vi "挥发酚断电保存全局变量.vi"() -> ()   [LabVIEW 2022 SP3, in "挥发酚.lvlib"]
panel:
  in  "数据时间":T1
  in  "维护模式":bool
  in  "校准信息":T2
  in  "校准信息改变":bool
  in  "关键参数改变":bool
  in  "标样核查自动补测":bool caption="通讯连接"
  in  "跨度核查自动补测":bool caption="通讯连接"
  in  "零点核查自动补测":bool caption="通讯连接"
  out "校准条件":cluster{"线性相关系数":dbl}={"线性相关系数"=0.99}
  in  "CODMn关键参数":T3={"测量量程"=0.0, "测量检出限"=0.0, "测量精度"=0.0, "测量间隔"=0.0, "消解温度"=95.0, "消解时长"=25.0, "三项式系数"=0.0, "二次多项式系数"=0.0, "曲线斜率"=0.0, "曲线截距"=0.0, "线性相关系数"=0.0, "空白校准时间"=timestamp(0 s since 1904-01-01), "标样校准时间"=timestamp(0 s since 1904-01-01), "测量信号值"=0.0, "稀释倍数"=0.0, "量程系数"=0.0}
  in  "CODMn仪器参数":T4
  in  "阀口名称":T5={"V"="试剂1", "V 2"="试剂2", "V 3"="试剂3", "V 4"="试剂4", "V 5"="试剂5", "V 6"="试剂6", "V 7"="试剂7", "V 8"="试剂8", "V 9"="试剂9", "V 10"="试剂10", "V 11"="试剂11", "V 12"="试剂12", "V9-1"="试剂13", "V9-2"="试剂14"}
  out "阀配置":u8(ring) items=["三通阀", "排阀"]
  in  "远程标样校准":enum16{"标液1", "标液2", "标液3", "标液4"}(ring)
  in  "远程校准量程":enum16{"低量程1", "低量程2", "高量程1", "高量程2"}(ring)
  in  "站号":u16(ring)=1 items=["挥发酚"=1, "总氮"=2, "氨氮"=3]
  out "公式、校准输出":T6={"公式"={"X^2"=0.0, "X"=nan, "B"=nan}, "校准"={"校准？"=FALSE, "校准点1-5"=0, "校准浓度"=0.0}}
  in  "MB通信方式选择":enum16{"串口", "TCP"}(ring)
  in  "PORT":string="502"
  in  "IP":string="192.168.1.203"
  in  "VISA Resource":refnum<visa-resource-name>="COM4"
  in  "运行周期":T7={"运行模式"=enum."维护模式", "质控频次"=enum."关闭", "空白核查时间"=2, "跨度核查时间"=6, "测量间隔"=240} {"跨度核查时间" items=["00H", "01H", "02H", "03H", "04H", "05H", "06H", "07H", "08H", "09H", "10H", "11H", "12H", "13H", "14H", "15H", "16H", "17H", "18H", "19H", "20H", "21H", "22H", "23H", "关闭"]; "空白核查时间" items=["00H", "01H", "02H", "03H", "04H", "05H", "06H", "07H", "08H", "09H", "10H", "11H", "12H", "13H", "14H", "15H", "16H", "17H", "18H", "19H", "20H", "21H", "22H", "23H", "关闭"]}
  in  "流程路径":path=path "C:/Users/std/Documents/斯坦道流程文件/流程.xml"
  in  "质控参数设置":T8 {"标准液标准偏差" format="%#_g%"; "跨度标准液偏差" format="%#_g%"}
  # "运行模式："
  # "质控频次："
  # "零点核查时间："
  # "跨度核查时间："
  # "测量间隔："
  # "质控参数设置"
  # "监测参数"
  # "CODMn"
  # "跨度值"
  # "零点核查标准液浓度"
  # "跨度核查标准液浓度"
  # "标样核查标准液浓度"
  # "零点核查标准液偏差"
  # "跨度核查标准液偏差"
  # "标样核查标准液偏差"
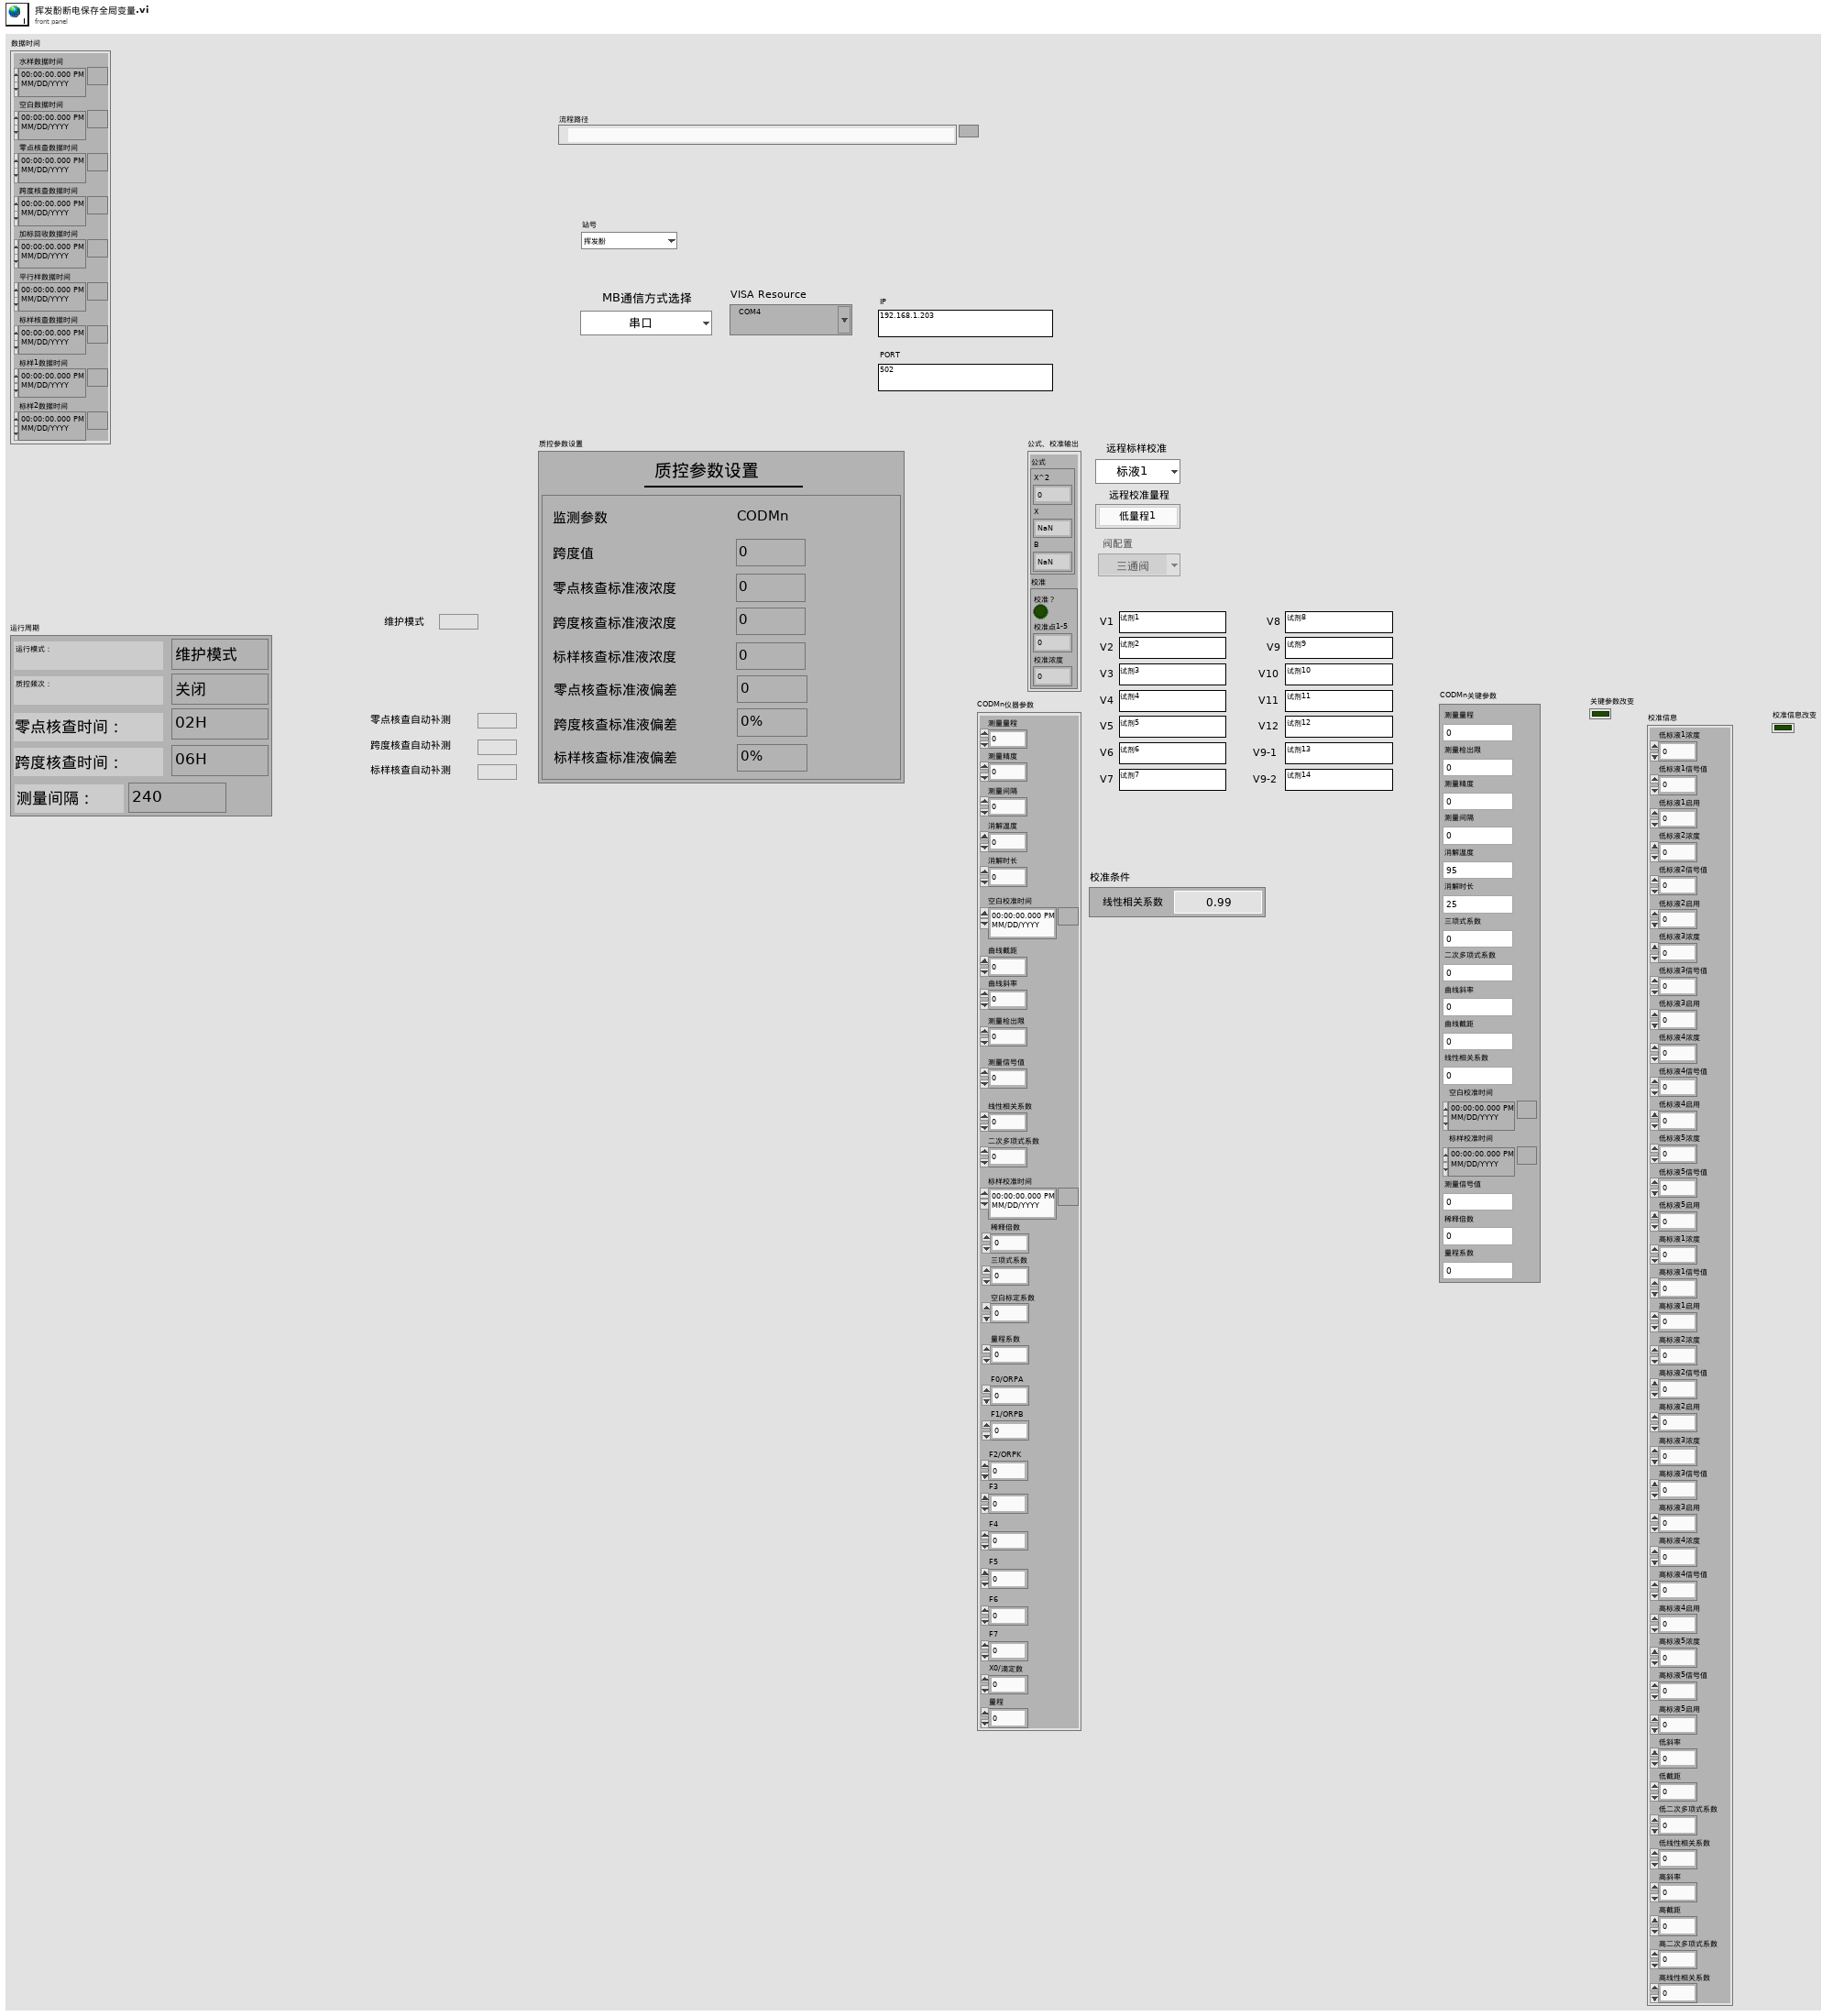
[diagram p1: front panel]
types:
  T1 = cluster{"水样数据时间":timestamp, "空白数据时间":timestamp, "零点核查数据时间":timestamp, "跨度核查数据时间":timestamp, "加标回收数据时间":timestamp, "平行样数据时间":timestamp, "标样核查数据时间":timestamp, "标样1数据时间":timestamp, "标样2数据时间":timestamp}
  T2 = cluster{"低标液1浓度":dbl, "低标液1信号值":dbl, "低标液1启用":u16, "低标液2浓度":dbl, "低标液2信号值":dbl, "低标液2启用":u16, "低标液3浓度":dbl, "低标液3信号值":dbl, "低标液3启用":u16, "低标液4浓度":dbl, "低标液4信号值":dbl, "低标液4启用":u16, "低标液5浓度":dbl, "低标液5信号值":dbl, "低标液5启用":u16, "高标液1浓度":dbl, "高标液1信号值":dbl, "高标液1启用":u16, "高标液2浓度":dbl, "高标液2信号值":dbl, "高标液2启用":u16, "高标液3浓度":dbl, "高标液3信号值":dbl, "高标液3启用":u16, "高标液4浓度":dbl, "高标液4信号值":dbl, "高标液4启用":u16, "高标液5浓度":dbl, "高标液5信号值":dbl, "高标液5启用":u16, "低斜率":dbl, "低截距":dbl, "低二次多项式系数":dbl, "低线性相关系数":dbl, "高斜率":dbl, "高截距":dbl, "高二次多项式系数":dbl, "高线性相关系数":dbl}
  T3 = cluster{"测量量程":sgl, "测量检出限":sgl, "测量精度":sgl, "测量间隔":sgl, "消解温度":sgl, "消解时长":sgl, "三项式系数":sgl, "二次多项式系数":sgl, "曲线斜率":sgl, "曲线截距":sgl, "线性相关系数":sgl, "空白校准时间":timestamp, "标样校准时间":timestamp, "测量信号值":sgl, "稀释倍数":sgl, "量程系数":sgl}
  T4 = cluster{"测量量程":dbl, "测量精度":dbl, "测量间隔":dbl, "消解温度":dbl, "消解时长":dbl, "空白校准时间":timestamp, "曲线截距":dbl, "曲线斜率":dbl, "测量检出限":dbl, "测量信号值":dbl, "线性相关系数":dbl, "二次多项式系数":dbl, "标样校准时间":timestamp, "稀释倍数":dbl, "三项式系数":dbl, "空白标定系数":dbl, "量程系数":dbl, "F0/ORPA":dbl, "F1/ORPB":dbl, "F2/ORPK":dbl, "F3":dbl, "F4":dbl, "F5":dbl, "F6":dbl, "F7":dbl, "X0/滴定数":dbl, "量程":dbl}
  T5 = cluster{"V":string, "V 2":string, "V 3":string, "V 4":string, "V 5":string, "V 6":string, "V 7":string, "V 8":string, "V 9":string, "V 10":string, "V 11":string, "V 12":string, "V9-1":string, "V9-2":string}
  T6 = cluster{"公式":cluster{"X^2":dbl, "X":dbl, "B":dbl}, "校准":cluster{"校准？":bool, "校准点1-5":u16, "校准浓度":dbl}}
  T7 = cluster{"运行模式":enum16{"维护模式", "常规模式", "应急模式", "质控模式", "性能测试"}, "质控频次":enum16{"关闭", "每天", "星期一", "星期二", "星期三", "星期四", "星期五", "星期六", "星期日"}, "空白核查时间":u16, "跨度核查时间":u16, "测量间隔":u16}
  T8 = cluster{"跨度值":dbl, "零点标准液浓度":dbl, "跨度标准液浓度":dbl, "标准液标准浓度":dbl, "零点标准液偏差":dbl, "跨度标准液偏差":dbl, "标准液标准偏差":dbl}
diagram:
